vi "FormatDate.vi"(2 "error in":errorcluster, 3 "time stamp":timestamp) -> (0 "error out":errorcluster, 1 "Date":string)   [LabVIEW 2018]
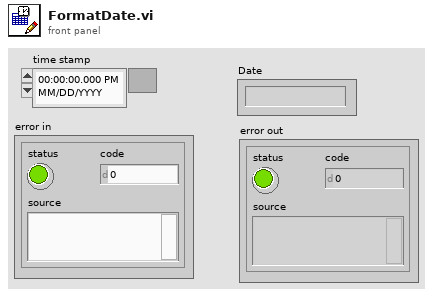
[diagram p1: front panel]
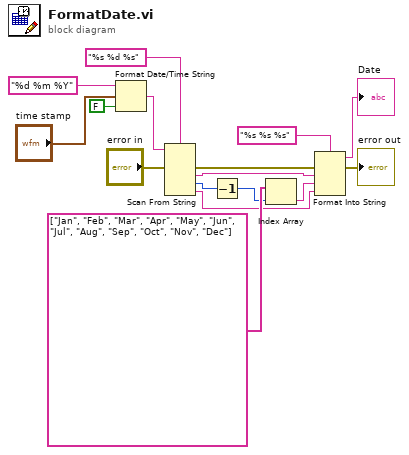
[diagram p0: block diagram]
diagram:
  n1 = Format Date/Time String(time format string (%c)="%d %m %Y", seconds (now)="time stamp", UTC format=FALSE) -> (date/time string=w14:string)
  n2 = Scan From String(format string="%s %d %s", input string=w14, error in="error in") -> (error out=w4:errorcluster, output 1=w7:string, output 2=w12:i32, output 3=w6:string)  [unwired: 4 in, 2 out]
  n3 = Decrement(x=w12) -> (x-1=w10:i32)
  n4 = Index Array(array=string[] ["Jan", "Feb", "Mar", "Apr", "May", "Jun", "Jul", "Aug", "Sep", "Oct", "Nov", "Dec"], index=w10) -> (element=w8:string)
  n5 = Format Into String(format string="%s %s %s", error in=w4, w7, w8, w6) -> (resulting string=→"Date":string, error out=→"error out":errorcluster)  [unwired: 1 in]
